vi "On Triggered Log State Change.vi"(8 "error in (no error)":errorcluster, 10 "Log State":T2, 11 "Trigger Event Registrations in":T1[](array[typedef])) -> (0 "error out":errorcluster, 3 "Trigger Event Registrations out":T1[](array[typedef]))   [LabVIEW 2015, in "Triggered Log.lvclass"]
doc: "Notify all registered listeners that the log has changed state. Send the new log state and the specifed User Data."
uses:
  Triggered Log.lvclass
  Triggered Log State Change Event Registration.ctl
  Triggered Log State.ctl
  Triggered Log State Change Event Data.ctl
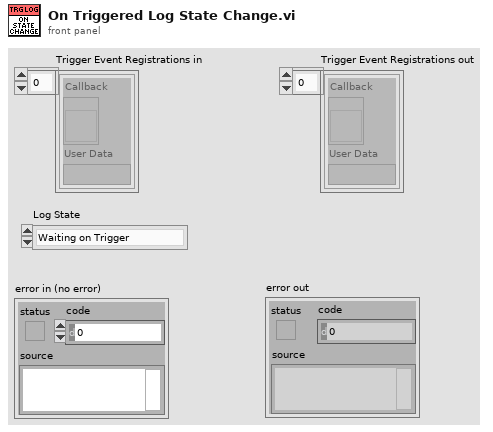
[diagram p1: front panel]
types:
  T1 = typedef "Triggered Log.lvclass/Triggered Log State Change Event Registration.ctl" = cluster{"Callback":refnum<vi>, "User Data":variant}
  T2 = typedef "Triggered Log.lvclass/Triggered Log State.ctl" = enum16{"Waiting on Trigger", "Triggered", "Posttrigger", "Complete", "Idle", "Error"}
  T3 = typedef "Triggered Log.lvclass/Triggered Log State Change Event Data.ctl" = cluster{"Log State":T2, "User Data":variant}
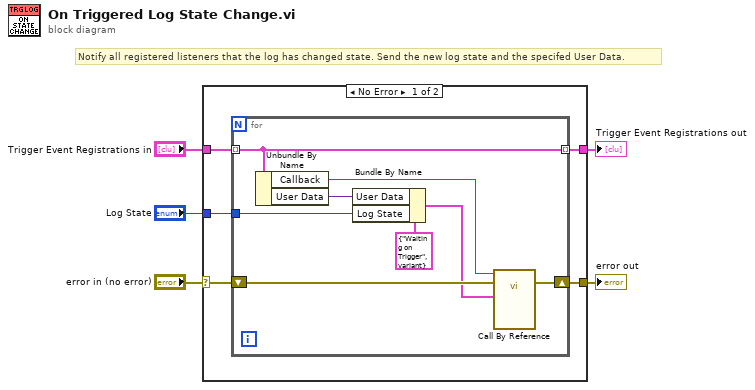
[diagram p0: block diagram]
diagram:
  # "Notify all registered listeners that the log has changed state. Send the new log state and the specifed User Data."
  n1 = case shown="No Error" "error in (no error)" {
    selector: "error in (no error)" -> [w6 w19]
    tunnel: "Trigger Event Registrations in" -> [w10 w20]
    tunnel: [w9 w19] -> w4
    tunnel: "Log State" -> [w8 _]
    tunnel: [w7 w20] -> w2
    frame No Error {
      n2 = for {
        tunnel: w10 -> [w11] mode=indexing
        shift-right: [w15] -> w9
        shift-left: w6 -> [w18]
        tunnel: w8 -> [w12]
        tunnel: [w11] -> w7 mode=indexing
        n3 = Unbundle By Name(w11) -> ("Callback"=w17:refnum<vi>, "User Data"=w16:variant)
        n4 = Bundle By Name(cluster=T3 {"Log State"=enum."Waiting on Trigger", "User Data"=variant} ("Trigger Event Data"), "User Data"=w16, "Log State"=w12) -> (w14:T3)
        n5 = call-by-ref "?"(reference=w17, error in=w18, "Log State Change Event Data"=w14) -> (error out=w15:errorcluster)  [unwired: 11 in, 1 out]
      }
    }
    frame Error {
    }
  }
  "error out" <- w4
  "Trigger Event Registrations out" <- w2
